vi "variant to datatype string.vi"(8 "error in (no error)":errorcluster, 10 "Variant":variant) -> (0 "error out":errorcluster, 2 "datatype string":string)   [LabVIEW 2016, in "FPGA Addon System Explorer.lvlib"]
uses:
  FPGA Addon System Explorer.lvlib
  <vilib>/Utility/Data Type/NI_Data Type.lvlib
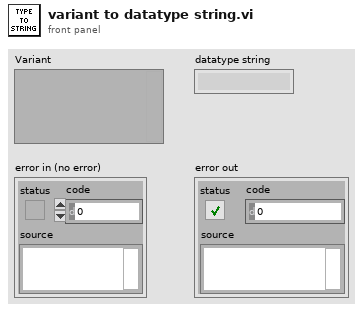
[diagram p1: front panel]
types:
  T1 = typedef "NI_Data Type.lvlib/Data Type.ctl" = enum8{"Invalid Type", "Void", "I8", "I16", "I32", "I64", "U8", "U16", "U32", "U64", "Single Float", "Double Float", "Extended Float", "Single Complex", "Double Complex", "Extended Complex", "Enum U8", "Enum U16", "Enum U32", "Enum U64", "Single Float With Unit", "Double Float With Unit", "Extended Float With Unit", "Single Complex with Unit", "Double Complex with Unit", "Extended Complex with Unit", "Boolean", "String", "Path", "Picture", "Tag", "Array", "Cluster", "Variant", "LV Variant", "Waveform", "Timestamp", "Digital Waveform", "Digital Data", "ExpressData", "Refnum", "External Data", "VI", "Poly VI", "LabVIEW Class Instance", "Fixed Point"}
  T2 = typedef "LVFixedPointRepRangeTypeDef.ctl" = cluster{"Range Min":dbl, "Range Max":dbl, "Delta":dbl}
  T3 = typedef "LVFixedPointRepBitsTypeDef.ctl" = cluster{"Signed":bool, "Word Length":u32, "Integer Word Length":i32}
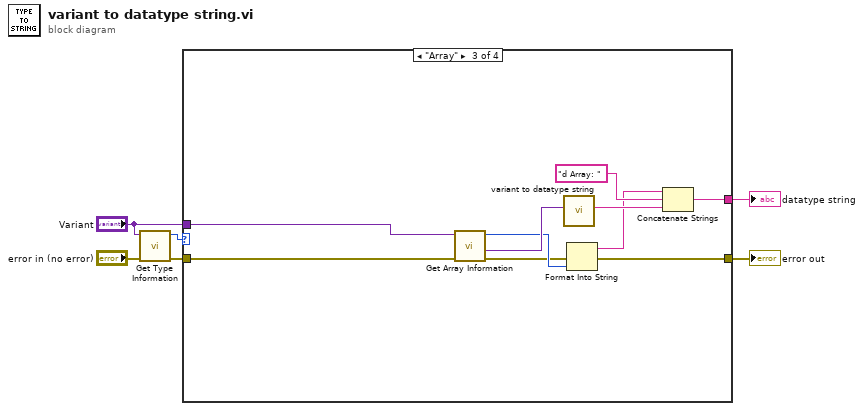
[diagram p0: block diagram]
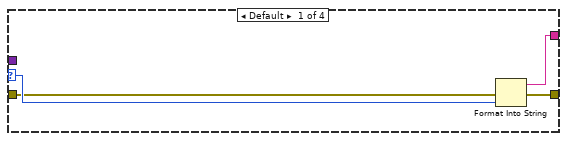
[diagram p2: hidden frame]
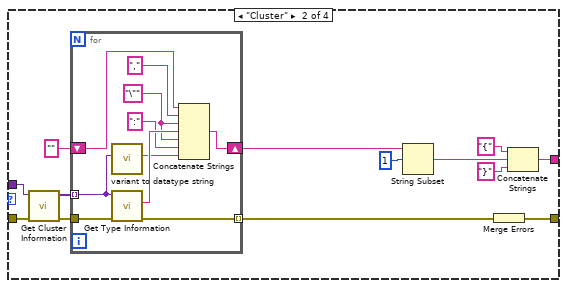
[diagram p3: hidden frame]
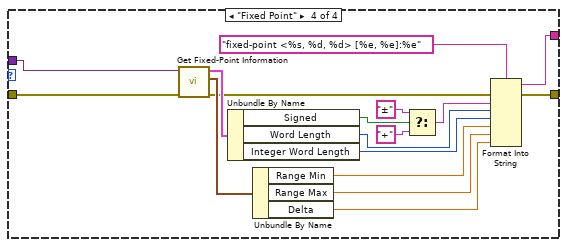
[diagram p4: hidden frame]
diagram:
  n1 = call <vilib>:"Get Type Information.vi"("error in (no error)"="error in (no error)", "Variant"="Variant") -> ("error out"=w2:errorcluster, "Type"=w6:T1)  [unwired: 5 in, 3 out]
  n2 = case shown="\"Array\"" w6 {
    selector: w6 -> [w10 _ _ _]
    tunnel: [w9 w15 w42 w47] -> w5
    tunnel: "Variant" -> [_ w23 w43 w60]
    tunnel: w2 -> [w8 w14 w36 w46]
    tunnel: [w7 w11 w34 w44] -> w1
    frame Default {
      n3 = Format Into String(error in=w8, w10) -> (resulting string=w9:string, error out=w7:errorcluster)  [unwired: 2 in]
    }
    frame "Cluster" {
      n4 = call <vilib>:"Get Cluster Information.vi"("error in (no error)"=w14, "Variant"=w23) -> ("error out"=w13:errorcluster, "Cluster Elements"=w22:variant[])  [unwired: 8 in]
      n5 = for {
        tunnel: w22 -> [w33] mode=indexing
        shift-right: [w26] -> w20
        shift-left: "" ("Name") -> [w28]
        tunnel: w13 -> [w25]
        tunnel: [w24] -> w12 mode=indexing
        w29 = "\"" ("Name")
        n6 = call "variant to datatype string.vi"("Variant"=w33) -> ("datatype string"=w30:string)  [unwired: 9 in, 1 out]
        n7 = call <vilib>:"Get Type Information.vi"("error in (no error)"=w25, "Variant"=w33) -> ("error out"=w24:errorcluster, "Name"=w32:string)  [unwired: 5 in, 3 out]
        n8 = Concatenate Strings(w28, "," ("string"), w29, w32, w29, ":" ("string"), w30) -> (w26:string)
      }
      n9 = String Subset(string=w20, offset (0)=1) -> (substring=w18:string)  [unwired: 1 in]
      n10 = Merge Errors(w12) -> (w11:errorcluster)
      n11 = Concatenate Strings("{" ("string"), w18, "}" ("string")) -> (w15:string)
    }
    frame "Array" {
      n12 = call <vilib>:"Get Array Information.vi"("error in (no error)"=w36, "Variant"=w43) -> ("error out"=w35:errorcluster, "Array Element Data Type"=w41:variant, "Number of Dimensions"=w38:i32)  [unwired: 6 in, 1 out]
      n13 = call "variant to datatype string.vi"("Variant"=w41) -> ("datatype string"=w40:string)  [unwired: 9 in, 1 out]
      n14 = Format Into String(error in=w35, w38) -> (resulting string=w37:string, error out=w34:errorcluster)  [unwired: 2 in]
      n15 = Concatenate Strings(w37, "d Array: " ("string"), w40) -> (w42:string)
    }
    frame "Fixed Point" {
      n16 = call <vilib>:"Get Fixed-Point Information.vi"("error in (no error)"=w46, "Variant"=w60) -> ("error out"=w45:errorcluster, "FXP Range"=w58:T2, "FXP Representation"=w59:T3)  [unwired: 6 in, 1 out]
      n17 = Unbundle By Name(w59) -> ("Signed"=w56:bool, "Word Length"=w52:u32, "Integer Word Length"=w51:i32)
      n18 = Unbundle By Name(w58) -> ("Range Min"=w50:dbl, "Range Max"=w49:dbl, "Delta"=w48:dbl)
      n19 = Select(t="±", s=w56, f="+") -> (s? t:f=w53:string)
      n20 = Format Into String(format string="fixed-point <%s, %d, %d> [%e, %e]:%e", error in=w45, w53, w52, w51, w50, w49, w48) -> (resulting string=w47:string, error out=w44:errorcluster)  [unwired: 1 in]
    }
  }
  "datatype string" <- w5
  "error out" <- w1
